vi "Write SQLite Connection.vi"(8 "error in (no error)":errorcluster, 10 "SQLite.lvlib:Connection":refnum<class "Connection.lvclass">, 11 "SQLite_API in":refnum<class "SQLite_API.lvclass">) -> (0 "error out":errorcluster, 3 "SQLite_API out":refnum<class "SQLite_API.lvclass">)   [LabVIEW 2021, in "SQLite_API.lvclass"]
uses:
  <userlib>/John_Lib/DataBase/SQLite_API/SQLite_API.lvclass
  <userlib>/John_Lib/DataBase/SQLite_API/SQLite_API.lvclass/SQLite_API.ctl
  <vilib>/drjdpowell/SQLite Library/SQL Connection/Connection.lvclass
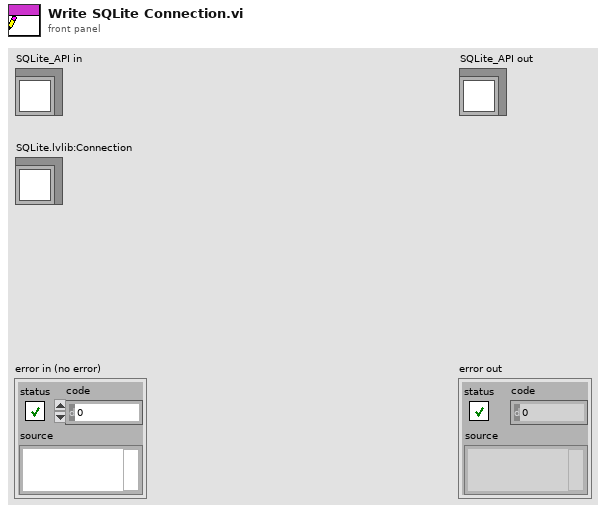
[diagram p1: front panel]
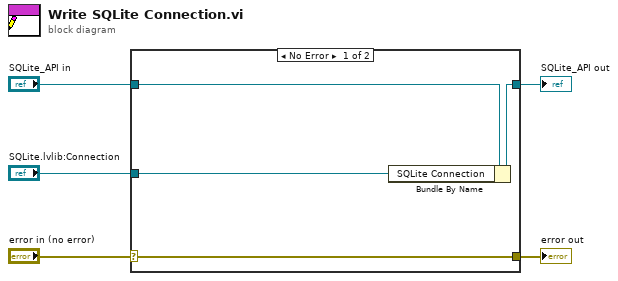
[diagram p0: block diagram]
diagram:
  n1 = case shown="No Error" "error in (no error)" {
    selector: "error in (no error)" -> [w9 w10]
    tunnel: [w9 w10] -> w4
    tunnel: [w7 w11] -> w2
    tunnel: "SQLite_API in" -> [w8 w11]
    tunnel: "SQLite.lvlib:Connection" -> [w6 _]
    frame No Error {
      n2 = Bundle By Name(cluster=w8, "SQLite Connection"=w6) -> (w7:refnum<class "SQLite_API.lvclass">)
    }
    frame Error {
    }
  }
  "error out" <- w4
  "SQLite_API out" <- w2
